vi "PM100D_Open.vi"(0 "VISA resource name":refnum<visa-resource-name>) -> (1 "VISA out":refnum<visa-resource-name>, 2 "Instrument":string, 3 "SN":string, 4 "error out":errorcluster)   [LabVIEW 2014]
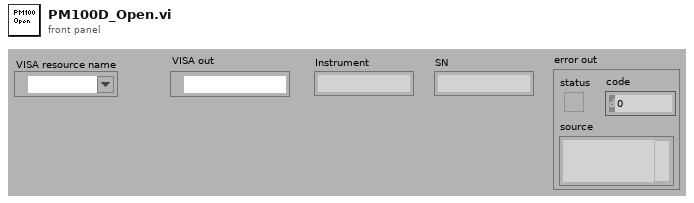
[diagram p1: front panel]
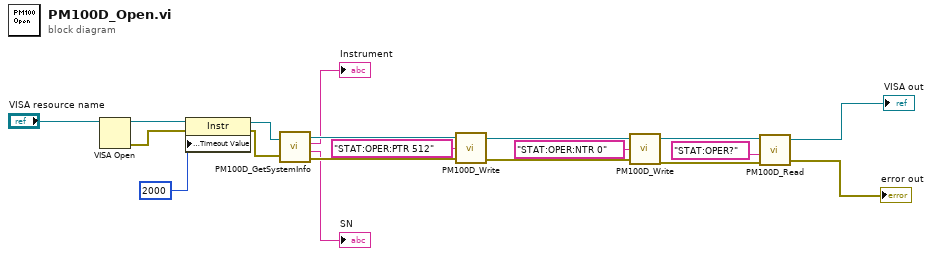
[diagram p0: block diagram]
diagram:
  n1 = VISA Open(VISA resource name="VISA resource name") -> (VISA resource name=w6:refnum<visa-resource-name>, error out=w1:errorcluster)  [unwired: 1 in, 3 out]
  n2 = property class="Instr"(reference=w6, error in=w1, "General Settings:Timeout Value"=u32 2000) -> (reference out=w7:refnum<visa-resource-name>, error out=w2:errorcluster)
  n3 = call "PM100D_GetSystemInfo.vi"("VISA in"=w7, "error in"=w2) -> ("VISA out"=w9:refnum<visa-resource-name>, "Instrument"=→"Instrument":string, "SN"=→"SN":string, "error out"=w11:errorcluster)
  n4 = call "PM100D_Write.vi"("error in (no error)"=w11, "Command"="STAT:OPER:PTR 512", "VISA in"=w9) -> ("error out"=w12:errorcluster, "VISA out"=w10:refnum<visa-resource-name>)
  n5 = call "PM100D_Write.vi"("error in (no error)"=w12, "Command"="STAT:OPER:NTR 0", "VISA in"=w10) -> ("error out"=w16:errorcluster, "VISA out"=w14:refnum<visa-resource-name>)
  n6 = call "PM100D_Read.vi"("error in (no error)"=w16, "Command"="STAT:OPER?", "VISA in"=w14) -> ("error out"=→"error out":errorcluster, "VISA out"=→"VISA out":refnum<visa-resource-name>)  [unwired: 1 in, 1 out]
